vi "readTelemetryHardpointData.vi"(8 "error in (no error)":errorcluster, 10 "Parser":refnum<class "U8ArrayParserAutoIndexing.lvclass">, 11 "M1M3SAL in":refnum<class "M1M3SAL.lvclass">) -> (0 "error out":errorcluster, 2 "EventSummaryState":variant, 3 "M1M3SAL out":refnum<class "M1M3SAL.lvclass">)   [LabVIEW 2016, in "M1M3SupportCommunicator.lvlib" / "M1M3SAL.lvclass"]
uses:
  M1M3SAL.lvclass
  Common_RT_Utilities/U8ArrayParserAutoIndexing/U8ArrayParserAutoIndexing.lvclass
  DataTypes/Topics/TelemetryHardpointData.ctl
  DataTypes/Topics/Parts/Timestamp.ctl
  DataTypes/Topics/M1M3SupportTopics.lvlib
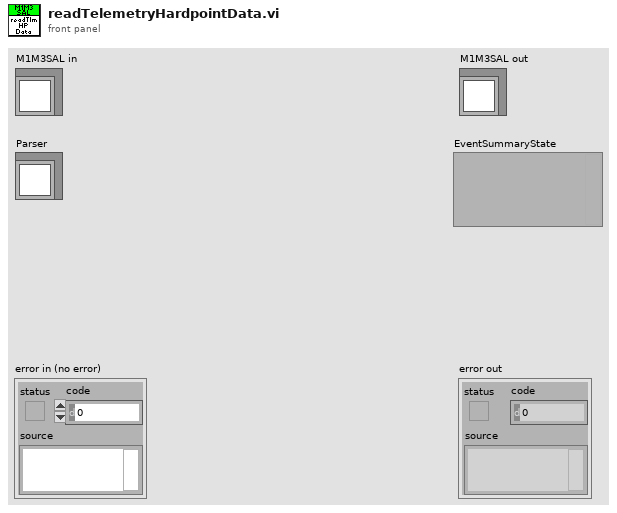
[diagram p1: front panel]
types:
  T1 = typedef "M1M3SupportTopics.lvlib/TelemetryHardpointData.ctl" = cluster{"Timestamp":T2, "StepsCommanded":i16[], "Force":sgl[], "Encoder":i32[], "ILCFault":bool[], "CWLimitOperated":bool[], "CCWLimitOperated":bool[], "BroadcastCounter":u8[]}
  T2 = typedef "M1M3SupportTopics.lvlib/Timestamp.ctl" = dbl
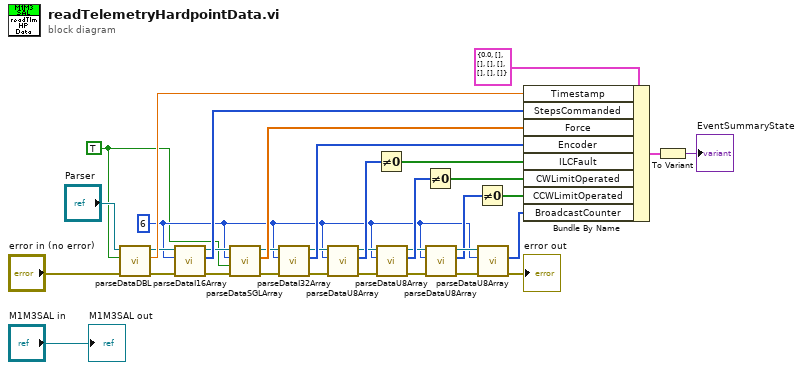
[diagram p0: block diagram]
diagram:
  w1 = TRUE ("OverrideSwapBytes")
  w2 = 6 ("Length")
  n1 = call "parseDataDBL.vi"("error in (no error)"="error in (no error)", "OverrideSwapBytes"=w1, "U8ArrayParserAutoIndexing in"="Parser") -> ("error out"=w19:errorcluster, "Data"=w29:dbl, "U8ArrayParserAutoIndexing out"=w20:refnum<class "U8ArrayParserAutoIndexing.lvclass">)  [unwired: 6 in]
  n2 = call "parseDataI16Array.vi"("U8ArrayParserAutoIndexing in"=w20, "Length"=w2, "error in (no error)"=w19) -> ("U8ArrayParserAutoIndexing out"=w10:refnum<class "U8ArrayParserAutoIndexing.lvclass">, "Data"=w18:i16[], "error out"=w6:errorcluster)  [unwired: 5 in]
  n3 = call "parseDataSGLArray.vi"("U8ArrayParserAutoIndexing in"=w10, "Length"=w2, "OverrideSwapBytes"=w1, "error in (no error)"=w6) -> ("U8ArrayParserAutoIndexing out"=w9:refnum<class "U8ArrayParserAutoIndexing.lvclass">, "Data"=w17:sgl[], "error out"=w5:errorcluster)  [unwired: 4 in]
  n4 = call "parseDataI32Array.vi"("U8ArrayParserAutoIndexing in"=w9, "Length"=w2, "error in (no error)"=w5) -> ("U8ArrayParserAutoIndexing out"=w8:refnum<class "U8ArrayParserAutoIndexing.lvclass">, "Data"=w11:i32[], "error out"=w4:errorcluster)  [unwired: 5 in]
  n5 = call "parseDataU8Array.vi"("U8ArrayParserAutoIndexing in"=w8, "Length"=w2, "error in (no error)"=w4) -> ("U8ArrayParserAutoIndexing out"=w7:refnum<class "U8ArrayParserAutoIndexing.lvclass">, "Data"=w13:u8[], "error out"=w3:errorcluster)  [unwired: 5 in]
  n6 = Not Equal To 0?(x=w13) -> (x != 0?=w12:bool[])
  n7 = call "parseDataU8Array.vi"("U8ArrayParserAutoIndexing in"=w7, "Length"=w2, "error in (no error)"=w3) -> ("U8ArrayParserAutoIndexing out"=w22:refnum<class "U8ArrayParserAutoIndexing.lvclass">, "Data"=w26:u8[], "error out"=w24:errorcluster)  [unwired: 5 in]
  n8 = Not Equal To 0?(x=w26) -> (x != 0?=w14:bool[])
  n9 = call "parseDataU8Array.vi"("U8ArrayParserAutoIndexing in"=w22, "Length"=w2, "error in (no error)"=w24) -> ("U8ArrayParserAutoIndexing out"=w28:refnum<class "U8ArrayParserAutoIndexing.lvclass">, "Data"=w25:u8[], "error out"=w27:errorcluster)  [unwired: 5 in]
  n10 = Not Equal To 0?(x=w25) -> (x != 0?=w15:bool[])
  n11 = call "parseDataU8Array.vi"("U8ArrayParserAutoIndexing in"=w28, "Length"=w2, "error in (no error)"=w27) -> ("Data"=w16:u8[], "error out"=→"error out":errorcluster)  [unwired: 5 in, 1 out]
  n12 = Bundle By Name(cluster=T1 {"Timestamp"=0.0, "StepsCommanded"=[], "Force"=[], "Encoder"=[], "ILCFault"=[], "CWLimitOperated"=[], "CCWLimitOperated"=[], "BroadcastCounter"=[]} ("TelemetryHardpointData"), "Timestamp"=w29, "StepsCommanded"=w18, "Force"=w17, "Encoder"=w11, "ILCFault"=w12, "CWLimitOperated"=w14, "CCWLimitOperated"=w15, "BroadcastCounter"=w16) -> (w33:T1)
  n13 = To Variant(anything=w33) -> (Variant=→"EventSummaryState":variant)
  "M1M3SAL out" <- "M1M3SAL in"
